vi "Compressed data.vi"() -> ()   [LabVIEW 2012]
panel:
  out "Array 2":dbl[](array[numeric])
  in  "ARRAY IN":dbl[](array[numeric])
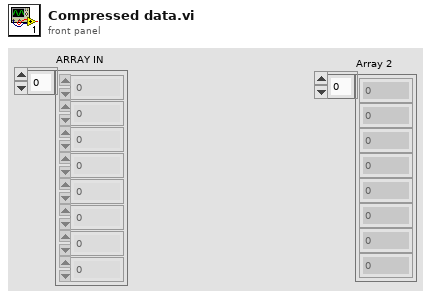
[diagram p1: front panel]
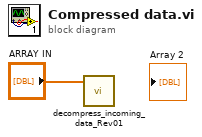
[diagram p0: block diagram]
diagram:
  n1 = call "decompress_incoming_data_Rev01.vi"("Input Data"="ARRAY IN") -> ()  [unwired: 9 in, 1 out]
